vi "Begin.vi"(11 "Image Size":T1=enum."160x120") -> (0 "error out":errorcluster)   [LabVIEW 2011]
doc: "Called before other user functions, this VI is expected to open initial I/O refnums, load in file data, and do all program initialization. Notice that the <B>error out</B> terminal is simply used for data flow. Wiring it to other structures or subVIs ensures that this VI runs first."
uses:
  <vilib>/Rock Robotics/WPI/Camera/WPI_CameraImageSize.ctl
  <vilib>/Rock Robotics/WPI/Camera/WPI_CameraWhite Balance Values.ctl
  <vilib>/Rock Robotics/WPI/Camera/WPI_CameraExposure Values.ctl
  <vilib>/Rock Robotics/WPI/Camera/WPI_CameraFrameRate.ctl
  <vilib>/Rock Robotics/SystemInterfaces/DIO/FPGA_DIOPWMChannel.ctl
  <vilib>/Rock Robotics/SystemInterfaces/Typedef/FPGA_TypedefDigitalModule.ctl
  <vilib>/Rock Robotics/SystemInterfaces/Typedef/FPGA_TypedefAnalogModule.ctl
  <vilib>/Rock Robotics/SystemInterfaces/AI/FPGA_AIChannel.ctl
  <vilib>/Rock Robotics/SystemInterfaces/DIO/FPGA_DIOChannel.ctl
  <vilib>/Rock Robotics/SystemInterfaces/DIO/FPGA_DIORelayChannel.ctl
  <vilib>/Rock Robotics/WPI/Joystick/WPI_JoystickDeviceEnum.ctl
  <vilib>/Rock Robotics/WPI/Relay/WPI_RelayDirection.ctl
  <vilib>/Rock Robotics/SystemInterfaces/Typedef/FPGA_TypedefSolenoidModule.ctl
  <vilib>/Rock Robotics/WPI/Solenoid/WPI_SolenoidChannel.ctl
  <vilib>/Rock Robotics/WPI/RobotDrive/WPI_RobotDriveOpen4MotorWithVictor.vi
  <vilib>/Rock Robotics/WPI/MotorControl/WPI_MotorControlOpen Victor.vi
  <vilib>/Rock Robotics/WPI/Counter/WPI_CounterDigitalInputToDigitalSource.vi
  <vilib>/Rock Robotics/WPI/Counter/WPI_CounterOpen Gear Tooth Sensor Mode.vi
  <vilib>/Rock Robotics/WPI/Solenoid/WPI_SolenoidOpenDouble.vi
  <vilib>/Rock Robotics/WPI/Compressor/WPI_CompressorGetSetRefNum.vi
  <vilib>/Rock Robotics/WPI/Encoder/WPI_EncoderType.ctl
panel:
  in  "Image Size 2":T1=enum."160x120"
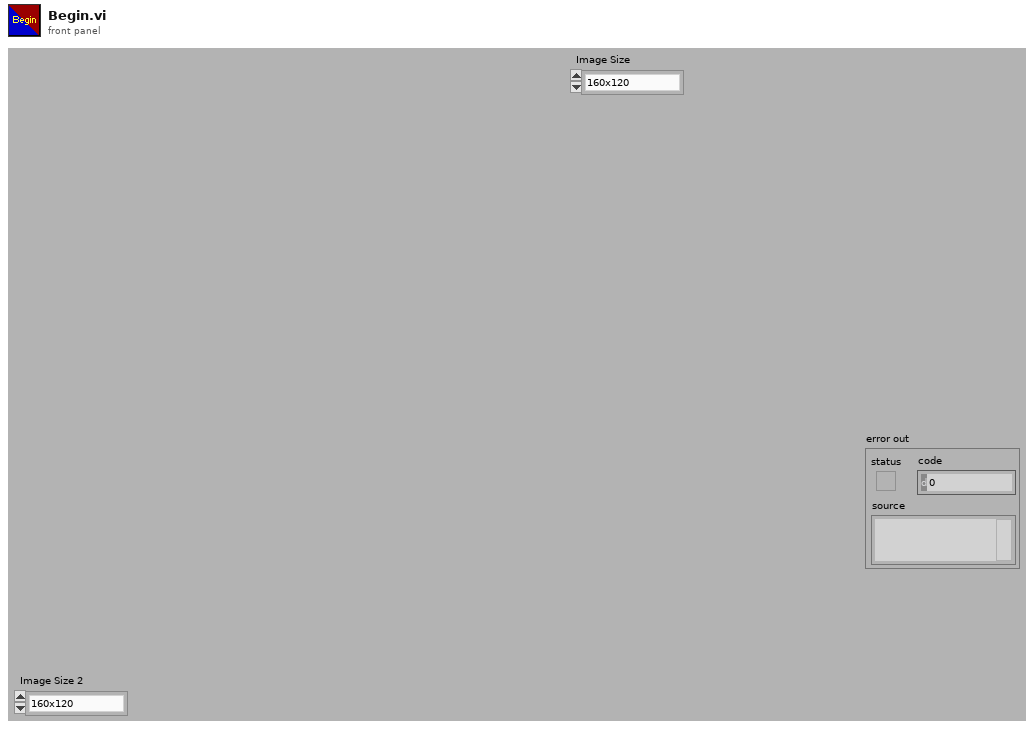
[diagram p1: front panel]
types:
  T1 = typedef "WPI_CameraImageSize.ctl" = enum16{"640x480", "320x240", "160x120"}
  T2 = typedef "FPGA_DIOChannel.ctl" = enum8{"DIO 1", "DIO 2", "DIO 3", "DIO 4", "DIO 5", "DIO 6", "DIO 7", "DIO 8", "DIO 9", "DIO 10", "DIO 11", "DIO 12", "DIO 13", "DIO 14", "Invalid"}
  T3 = typedef "FPGA_TypedefDigitalModule.ctl" = enum16{"Digital Module 1", "Digital Module 2"}
  T4 = typedef "WPI_RelayDirection.ctl" = enum16{"Both directions", "Forward only", "Reverse only"}
  T5 = typedef "FPGA_DIORelayChannel.ctl" = enum8{"Relay 1", "Relay 2", "Relay 3", "Relay 4", "Relay 5", "Relay 6", "Relay 7", "Relay 8", "Invalid"}
  T6 = typedef "WPI_SolenoidChannel.ctl" = enum8{"Solenoid 1", "Solenoid 2", "Solenoid 3", "Solenoid 4", "Solenoid 5", "Solenoid 6", "Solenoid 7", "Solenoid 8", "Invalid"}
  T7 = typedef "FPGA_TypedefSolenoidModule.ctl" = enum16{"Solenoid Module 1", "Solenoid Module 2"}
  T8 = typedef "WPI_JoystickDeviceEnum.ctl" = enum16{"USB 1", "USB 2", "USB 3", "USB 4", "Kinect 1", "Kinect 2"}
  T9 = typedef "FPGA_DIOPWMChannel.ctl" = enum8{"PWM 1", "PWM 2", "PWM 3", "PWM 4", "PWM 5", "PWM 6", "PWM 7", "PWM 8", "PWM 9", "PWM 10", "Invalid"}
  T10 = typedef "FPGA_AIChannel.ctl" = enum8{"AI 1", "AI 2", "AI 3", "AI 4", "AI 5", "AI 6", "AI 7", "AI 8", "Invalid"}
  T11 = typedef "FPGA_TypedefAnalogModule.ctl" = enum16{"Analog Module 1", "Analog Module 2"}
  T12 = typedef "WPI_CameraFrameRate.ctl" = u32
  T13 = typedef "WPI_CameraExposure Values.ctl" = enum16{"Auto", "Flicker-free 50 Hz", "Flicker-free 60 Hz", "Hold current"}
  T14 = typedef "WPI_CameraWhite Balance Values.ctl" = enum16{"Auto", "Fixed indoor", "Fixed outdoor 1", "Fixed outdoor 2", "Fixed fluorescent 1", "Fixed fluorescent 2", "Hold current"}
  T15 = typedef "WPI_MotorControlDeviceRef.ctl" = cluster{"DeviceStatus":errorcluster, "Type":enum16{"PWM", "CAN"}, "PWM":cluster{"Digital Module":T3, "PWM Channel":T9, "DeadBand":T16}, "CAN":cluster{"Device Number":u8, "Control Mode":T17, "Semaphore":T18, "Max Vout":dbl}, "Invert":bool, "TransformRef":T19, "InvTransformRef":T19}
  T16 = typedef "WPI_PWMDeadband.ctl" = cluster{"Name":string, "maxPositivePwm":i32, "minPositivePwm":i32, "centerPwm":i32, "maxNegativePwm":i32, "minNegativePwm":i32, "angularRange":u16}
  T17 = typedef "WPI_CANJaguar_ControlMode.ctl" = enum8{"Percent VBus", "Current", "Speed", "Position", "Voltage"}
  T18 = typedef "Semaphore RefNum" = refnum<k1>
  T19 = typedef "WPI_PWMTransform_ConPane.ctl" = refnum<vi>
  T20 = typedef "WPI_RobotDriveDevRef.ctl" = cluster{"DevStatus":errorcluster, "Motors[]":T15[], "Square Inputs":bool, "Max Output":dbl, "Isochronous":bool}
  T21 = typedef "WPI_CameraDevRef.ctl" = cluster{"Camera Address":string, "CameraStatus":errorcluster, "Acquire Image Notifier":refnum<notifier>}
  T22 = typedef "WPI_EncoderType.ctl" = enum16{"1x", "2x", "4x"}
  T23 = typedef "WPI_DigitalInputDevRef.ctl" = cluster{"DevStatus":errorcluster, "DIO Channel":T2, "Digital Module":T3}
  T24 = typedef "FPGA_CounterEncoderSourceConvertionLVSourceType.ctl" = cluster{"DevStatus":errorcluster, "AnalogTriggerMode?":bool, "DigitalMode":cluster{"Digital Module":T3, "DIO Channel":T25}, "AnalogTriggerMode":cluster{"AnalogTriggerIndex":T26, "OutputType":T27}}
  T25 = typedef "FPGA_DIODigitalSourceChannel.ctl" = enum8{"DIO 1", "DIO 2", "DIO 3", "DIO 4", "DIO 5", "DIO 6", "DIO 7", "DIO 8", "DIO 9", "DIO 10", "DIO 11", "DIO 12", "DIO 13", "DIO 14", "Disabled"}
  T26 = typedef "FPGA_AnalogTriggerIndex.ctl" = enum8{"Trig 0", "Trig 1", "Trig 2", "Trig 3", "Trig 4", "Trig 5", "Trig 6", "Trig 7", "Invalid"}
  T27 = typedef "FPGA_AnalogTriggerOutType.ctl" = enum16{"InWindow", "TriggerState", "Rising", "Falling"}
  T28 = typedef "WPI_EncoderDevRef.ctl" = cluster{"DevStatus":errorcluster, "EncoderIndex":T29, "CounterIndex":T30, "DistancePerCount":dbl, "Decoding Type":T22}
  T29 = typedef "FPGA_EncoderIdx.ctl" = enum8{"Enc 0", "Enc 1", "Enc 2", "Enc 3", "Invalid"}
  T30 = typedef "FPGA_CounterCtrSystemIndex.ctl" = enum8{"Ctr 0", "Ctr 1", "Ctr 2", "Ctr 3", "Ctr 4", "Ctr 5", "Ctr 6", "Ctr 7", "Invalid"}
  T31 = typedef "WPI_JoystickDevRef.ctl" = cluster{"Device":T8}
  T32 = typedef "WPI_AnalogChannelDevRef.ctl" = cluster{"DevStatus":errorcluster, "Analog Module":T11, "Analog Channel":T10}
  T33 = typedef "WPI_RelayDevRef.ctl" = cluster{"DevStatus":errorcluster, "Relay Channel":T5, "Digital Module":T3, "Relay Direction":T4}
  T34 = typedef "WPI_SolenoidDevRef.ctl" = cluster{"DevStatus":errorcluster, "Solenoid Module":T7, "Forward Solenoid Channel":T6, "Reverse Solenoid Channel":T6}
  T35 = typedef "WPI_CompressorDevRef.ctl" = cluster{"DevStatus":errorcluster, "DigitalInputDevRef":T23, "RelayDevRef":T33}
  T36 = typedef "WPI_CounterDevRef.ctl" = cluster{"DevStatus":errorcluster, "CntIndex":T30}
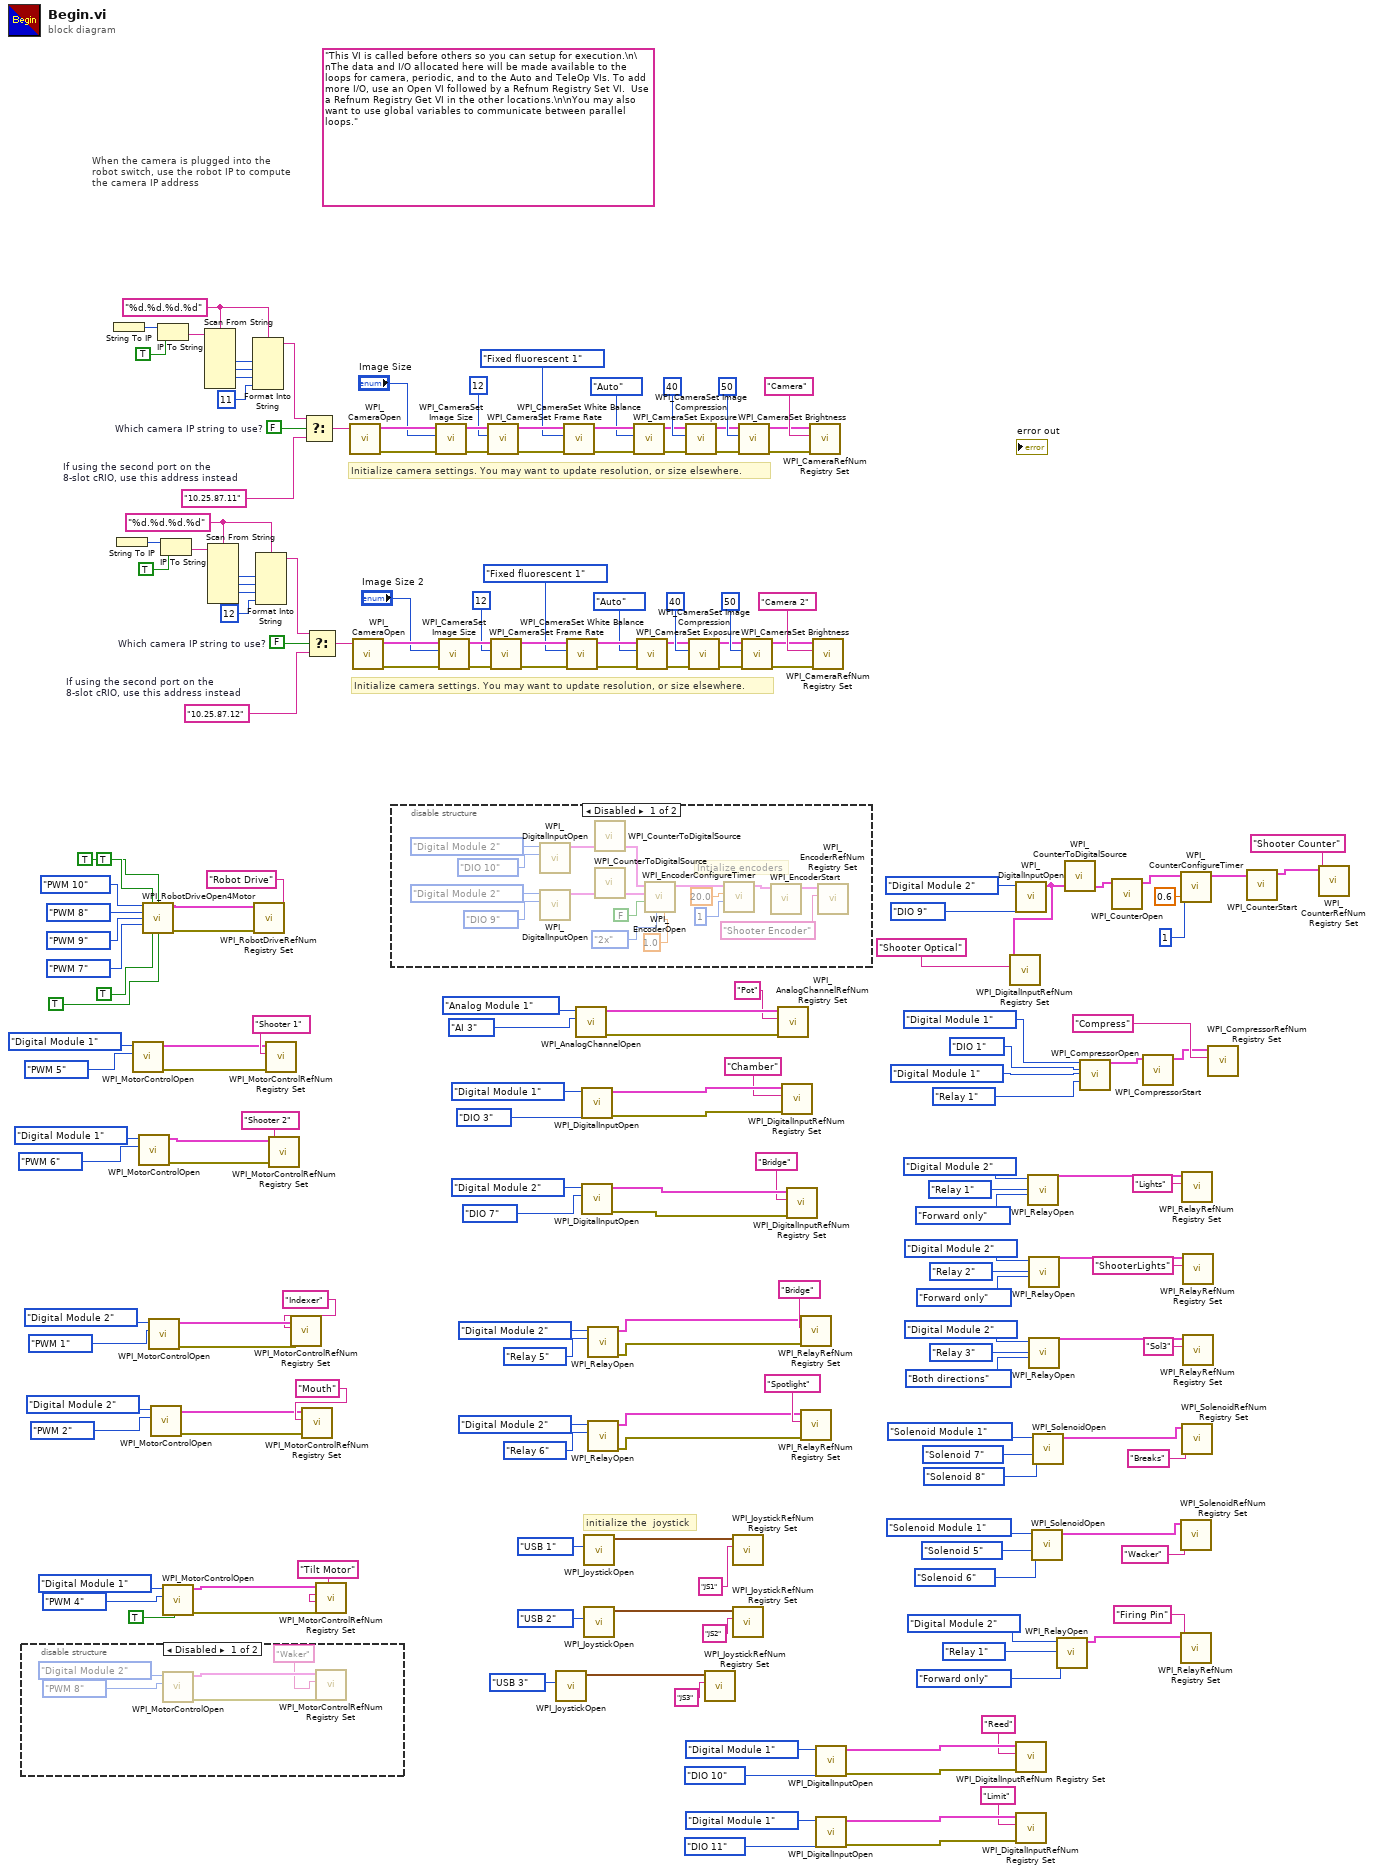
[diagram p0: block diagram]
diagram:
  w130 = FALSE  # Which camera IP string to use?
  w134 = "%d.%d.%d.%d" ("format string")
  w131 = "10.25.87.12"  # If using the second port on the 8-slot cRIO, use this address instead
  w163 = FALSE  # Which camera IP string to use?
  w167 = "%d.%d.%d.%d" ("format string")
  (unwired) "This VI is called before others so you can setup for execution.\n\nThe data and I/O allocated here will be made available to the loops for camera, periodic, and to the Auto and TeleOp VIs. To add more I/O, use an Open VI followed by a Refnum Registry Set VI.  Use a Refnum Registry Get VI in the other locations.\n\nYou may also want to use global variables to communicate between parallel loops."
  w164 = "10.25.87.11"  # If using the second port on the 8-slot cRIO, use this address instead
  # "initialize the  joystick"
  # "Initialize camera settings. You may want to update resolution, or size elsewhere."
  # "When the camera is plugged into the\nrobot switch, use the robot IP to compute\nthe camera IP address"
  # "Initialize camera settings. You may want to update resolution, or size elsewhere."
  n1 = disable-structure shown="Disabled" {
    frame Disabled {
      n2 = call-poly <vilib>:"WPI_MotorControlOpen.vi"("PWM Channel"=FPGA_DIOPWMChannel."PWM 8", "Digital Module (Module 1)"=FPGA_TypedefDigitalModule."Digital Module 2") -> ("error out"=w200:errorcluster, "MotorControlDeviceRef"=w199:T15)  [unwired: 8 in]
      n3 = call <vilib>:"WPI_MotorControlRefNum Registry Set.vi"("error in (no error)"=w200, "refnum name"="Waker", "MotorControlDevRef"=w199) -> ()  [unwired: 7 in, 2 out]
    }
    frame Enabled {
    }
  }
  n4 = String To IP() -> (0:w174:u32)  [unwired: 1 in]
  n5 = String To IP() -> (0:w141:u32)  [unwired: 1 in]
  n6 = call-poly <vilib>:"WPI_MotorControlOpen.vi"("PWM Channel"=FPGA_DIOPWMChannel."PWM 5", "Digital Module (Module 1)"=FPGA_TypedefDigitalModule."Digital Module 1") -> ("error out"=w113:errorcluster, "MotorControlDeviceRef"=w114:T15)  [unwired: 8 in]
  n7 = call-poly <vilib>:"WPI_MotorControlOpen.vi"("PWM Channel"=FPGA_DIOPWMChannel."PWM 6", "Digital Module (Module 1)"=FPGA_TypedefDigitalModule."Digital Module 1") -> ("error out"=w111:errorcluster, "MotorControlDeviceRef"=w112:T15)  [unwired: 8 in]
  n8 = call-poly <vilib>:"WPI_RobotDriveOpen4Motor.vi"("Rear Left Motor"=FPGA_DIOPWMChannel."PWM 10", "Rear Left Motor Inverted"=TRUE, "Rear Right Motor Inverted"=TRUE, "Rear Right Motor"=FPGA_DIOPWMChannel."PWM 8", "Front Left Motor"=FPGA_DIOPWMChannel."PWM 9", "Front Right Motor"=FPGA_DIOPWMChannel."PWM 7", "Front Left Motor Inverted"=TRUE, "Front Right Motor Inverted"=TRUE) -> ("RobotDriveDevRef"=w73:T20, "error out"=w72:errorcluster)  [unwired: 6 in]
  n9 = call-poly <vilib>:"WPI_MotorControlOpen.vi"("PWM Channel"=FPGA_DIOPWMChannel."PWM 1", "Digital Module (Module 1)"=FPGA_TypedefDigitalModule."Digital Module 2") -> ("error out"=w81:errorcluster, "MotorControlDeviceRef"=w82:T15)  [unwired: 8 in]
  n10 = call-poly <vilib>:"WPI_MotorControlOpen.vi"("PWM Channel"=FPGA_DIOPWMChannel."PWM 2", "Digital Module (Module 1)"=FPGA_TypedefDigitalModule."Digital Module 2") -> ("error out"=w106:errorcluster, "MotorControlDeviceRef"=w107:T15)  [unwired: 8 in]
  n11 = IP To String(1:TRUE ("dot notation? (F)"), 2:w174) -> (0:w172:string)
  n12 = IP To String(1:TRUE ("dot notation? (F)"), 2:w141) -> (0:w139:string)
  n13 = call-poly <vilib>:"WPI_MotorControlOpen.vi"("Invert"=TRUE, "PWM Channel"=FPGA_DIOPWMChannel."PWM 4", "Digital Module (Module 1)"=FPGA_TypedefDigitalModule."Digital Module 1") -> ("error out"=w100:errorcluster, "MotorControlDeviceRef"=w101:T15)  [unwired: 7 in]
  n14 = Scan From String(format string=w167, input string=w172) -> (output 1=w171:i32, output 2=w170:i32, output 3=w169:i32)  [unwired: 7 in, 3 out]
  n15 = Scan From String(format string=w134, input string=w139) -> (output 1=w138:i32, output 2=w137:i32, output 3=w136:i32)  [unwired: 7 in, 3 out]
  n16 = Format Into String(format string=w167, w171, w170, w169, 11 ("Compression")) -> (resulting string=w165:string)  [unwired: 2 in, 1 out]
  n17 = call <vilib>:"WPI_RobotDriveRefNum Registry Set.vi"("error in (no error)"=w72, "refnum name"="Robot Drive", "RobotDriveDevRef"=w73) -> ()  [unwired: 7 in, 2 out]
  n18 = Format Into String(format string=w134, w138, w137, w136, 12 ("Compression")) -> (resulting string=w132:string)  [unwired: 2 in, 1 out]
  n19 = call <vilib>:"WPI_MotorControlRefNum Registry Set.vi"("error in (no error)"=w113, "refnum name"="Shooter 1", "MotorControlDevRef"=w114) -> ()  [unwired: 7 in, 2 out]
  n20 = call <vilib>:"WPI_MotorControlRefNum Registry Set.vi"("error in (no error)"=w111, "refnum name"="Shooter 2", "MotorControlDevRef"=w112) -> ()  [unwired: 7 in, 2 out]
  n21 = call <vilib>:"WPI_MotorControlRefNum Registry Set.vi"("error in (no error)"=w81, "refnum name"="Indexer", "MotorControlDevRef"=w82) -> ()  [unwired: 7 in, 2 out]
  n22 = call <vilib>:"WPI_MotorControlRefNum Registry Set.vi"("error in (no error)"=w106, "refnum name"="Mouth", "MotorControlDevRef"=w107) -> ()  [unwired: 7 in, 2 out]
  n23 = Select(t=w165, s=w163, f=w164) -> (s? t:f=w166:string)
  n24 = Select(t=w132, s=w130, f=w131) -> (s? t:f=w133:string)
  n25 = call <vilib>:"WPI_MotorControlRefNum Registry Set.vi"("error in (no error)"=w100, "refnum name"="Tilt Motor", "MotorControlDevRef"=w101) -> ()  [unwired: 7 in, 2 out]
  n26 = call <vilib>:"WPI_CameraOpen.vi"("Camera Address"=w166) -> ("error out"=w186:errorcluster, "CameraDevRef"=w187:T21)  [unwired: 1 in, 8 out]
  n27 = call <vilib>:"WPI_CameraOpen.vi"("Camera Address"=w133) -> ("error out"=w153:errorcluster, "CameraDevRef"=w154:T21)  [unwired: 1 in, 8 out]
  n28 = disable-structure shown="Disabled" {
    frame Disabled {
      # "Intialize encoders"
      n29 = call <vilib>:"WPI_DigitalInputOpen.vi"("DIO Channel"=FPGA_DIOChannel."DIO 10", "Digital Module (Module 1)"=FPGA_TypedefDigitalModule."Digital Module 2") -> ("DigitalInputDevRef"=w215:T23)  [unwired: 8 in, 1 out]
      n30 = call <vilib>:"WPI_DigitalInputOpen.vi"("DIO Channel"=FPGA_DIOChannel."DIO 9", "Digital Module (Module 1)"=FPGA_TypedefDigitalModule."Digital Module 2") -> ("DigitalInputDevRef"=w211:T23)  [unwired: 8 in, 1 out]
      n31 = call-poly <vilib>:"WPI_CounterToDigitalSource.vi"("DigitalInputDevRef"=w215) -> ("Digital Source"=w214:T24)  [unwired: 6 in]
      n32 = call-poly <vilib>:"WPI_CounterToDigitalSource.vi"("DigitalInputDevRef"=w211) -> ("Digital Source"=w210:T24)  [unwired: 6 in]
      n33 = call <vilib>:"WPI_EncoderOpen.vi"("DistancePerCount"=1.0, "Decoding Type"=WPI_EncoderType."2x", "Invert Direction (False)"=FALSE, "BSource"=w210, "ASource"=w214) -> ("EncoderDevRef"=w208:T28)  [unwired: 5 in, 1 out]
      n34 = call <vilib>:"WPI_EncoderConfigureTimer.vi"("Number Samples to Average"=u8 1, "Minimum Rate"=20.0, "EncoderDevRef"=w208) -> ("EncoderDevRef"=w202:T28)  [unwired: 7 in, 1 out]
      n35 = call <vilib>:"WPI_EncoderStart.vi"("EncoderDevRef"=w202) -> ("EncoderDevRef"=w201:T28)  [unwired: 9 in, 1 out]
      n36 = call <vilib>:"WPI_EncoderRefNum Registry Set.vi"("refnum name"="Shooter Encoder", "EncoderDevRef"=w201) -> ()  [unwired: 8 in, 2 out]
    }
    frame Enabled {
    }
  }
  n37 = call <vilib>:"WPI_CameraSet Image Size.vi"("error in (no error)"=w186, "Image Size"="Image Size", "CameraDevRef"=w187) -> ("error out"=w185:errorcluster, "CameraDevRef Out"=w188:T21)  [unwired: 7 out]
  n38 = call <vilib>:"WPI_CameraSet Image Size.vi"("error in (no error)"=w153, "Image Size"="Image Size 2", "CameraDevRef"=w154) -> ("error out"=w152:errorcluster, "CameraDevRef Out"=w155:T21)  [unwired: 7 out]
  n39 = call <vilib>:"WPI_CameraSet Frame Rate.vi"("error in (no error)"=w185, "Frame Rate (fps)"=T12 12, "CameraDevRef"=w188) -> ("error out"=w184:errorcluster, "CameraDevRef Out"=w190:T21)  [unwired: 7 out]
  n40 = call <vilib>:"WPI_CameraSet Frame Rate.vi"("error in (no error)"=w152, "Frame Rate (fps)"=T12 12, "CameraDevRef"=w155) -> ("error out"=w151:errorcluster, "CameraDevRef Out"=w157:T21)  [unwired: 7 out]
  n41 = call <vilib>:"WPI_JoystickOpen.vi"("JoystickDevice"=WPI_JoystickDeviceEnum."USB 3") -> ("JoystickDevRef"=w50:T31)  [unwired: 10 out]
  n42 = call <vilib>:"WPI_CameraSet White Balance.vi"("error in (no error)"=w184, "White Balance"=WPI_CameraWhite_Balance_Values."Fixed fluorescent 1", "CameraDevRef"=w190) -> ("error out"=w183:errorcluster, "CameraDevRef Out"=w189:T21)  [unwired: 7 out]
  n43 = call <vilib>:"WPI_CameraSet White Balance.vi"("error in (no error)"=w151, "White Balance"=WPI_CameraWhite_Balance_Values."Fixed fluorescent 1", "CameraDevRef"=w157) -> ("error out"=w150:errorcluster, "CameraDevRef Out"=w156:T21)  [unwired: 7 out]
  n44 = call <vilib>:"WPI_AnalogChannelOpen.vi"("Analog Channel"=FPGA_AIChannel."AI 3", "Analog Module (Module 1)"=FPGA_TypedefAnalogModule."Analog Module 1") -> ("error out"=w95:errorcluster, "AIDeviceRef"=w97:T32)  [unwired: 8 in]
  n45 = call <vilib>:"WPI_DigitalInputOpen.vi"("DIO Channel"=FPGA_DIOChannel."DIO 3", "Digital Module (Module 1)"=FPGA_TypedefDigitalModule."Digital Module 1") -> ("error out"=w90:errorcluster, "DigitalInputDevRef"=w92:T23)  [unwired: 8 in]
  n46 = call <vilib>:"WPI_DigitalInputOpen.vi"("DIO Channel"=FPGA_DIOChannel."DIO 7", "Digital Module (Module 1)"=FPGA_TypedefDigitalModule."Digital Module 2") -> ("error out"=w62:errorcluster, "DigitalInputDevRef"=w64:T23)  [unwired: 8 in]
  n47 = call <vilib>:"WPI_JoystickOpen.vi"("JoystickDevice"=WPI_JoystickDeviceEnum."USB 1") -> ("JoystickDevRef"=w77:T31)  [unwired: 10 out]
  n48 = call <vilib>:"WPI_JoystickOpen.vi"("JoystickDevice"=WPI_JoystickDeviceEnum."USB 2") -> ("JoystickDevRef"=w76:T31)  [unwired: 10 out]
  n49 = call <vilib>:"WPI_RelayOpen.vi"("Relay Channel"=FPGA_DIORelayChannel."Relay 5", "Digital Module (Module 1)"=FPGA_TypedefDigitalModule."Digital Module 2") -> ("error out"=w67:errorcluster, "RelayDevRef"=w68:T33)  [unwired: 8 in]
  n50 = call <vilib>:"WPI_RelayOpen.vi"("Relay Channel"=FPGA_DIORelayChannel."Relay 6", "Digital Module (Module 1)"=FPGA_TypedefDigitalModule."Digital Module 2") -> ("error out"=w85:errorcluster, "RelayDevRef"=w86:T33)  [unwired: 8 in]
  n51 = call <vilib>:"WPI_CameraSet Exposure.vi"("error in (no error)"=w183, "Exposure"=WPI_CameraExposure_Values."Auto", "CameraDevRef"=w189) -> ("error out"=w182:errorcluster, "CameraDevRef Out"=w192:T21)  [unwired: 7 out]
  n52 = call <vilib>:"WPI_CameraSet Exposure.vi"("error in (no error)"=w150, "Exposure"=WPI_CameraExposure_Values."Auto", "CameraDevRef"=w156) -> ("error out"=w149:errorcluster, "CameraDevRef Out"=w159:T21)  [unwired: 7 out]
  n53 = call <vilib>:"WPI_CameraSet Image Compression.vi"("error in (no error)"=w182, "Compression"=40, "CameraDevRef"=w192) -> ("error out"=w181:errorcluster, "CameraDevRef Out"=w191:T21)  [unwired: 7 out]
  n54 = call <vilib>:"WPI_CameraSet Image Compression.vi"("error in (no error)"=w149, "Compression"=40, "CameraDevRef"=w159) -> ("error out"=w148:errorcluster, "CameraDevRef Out"=w158:T21)  [unwired: 7 out]
  n55 = call <vilib>:"WPI_JoystickRefNum Registry Set.vi"("refnum name"="JS3", "JoystickDevRef"=w50) -> ()  [unwired: 1 in, 9 out]
  n56 = call <vilib>:"WPI_JoystickRefNum Registry Set.vi"("refnum name"="JS1", "JoystickDevRef"=w77) -> ()  [unwired: 1 in, 9 out]
  n57 = call <vilib>:"WPI_JoystickRefNum Registry Set.vi"("refnum name"="JS2", "JoystickDevRef"=w76) -> ()  [unwired: 1 in, 9 out]
  n58 = call <vilib>:"WPI_CameraSet Brightness.vi"("error in (no error)"=w181, "Brightness"=50, "CameraDevRef"=w191) -> ("error out"=w179:errorcluster, "CameraDevRef Out"=w180:T21)  [unwired: 7 out]
  n59 = call <vilib>:"WPI_CameraSet Brightness.vi"("error in (no error)"=w148, "Brightness"=50, "CameraDevRef"=w158) -> ("error out"=w146:errorcluster, "CameraDevRef Out"=w147:T21)  [unwired: 7 out]
  n60 = call <vilib>:"WPI_AnalogChannelRefNum Registry Set.vi"("error in (no error)"=w95, "refnum name"="Pot", "AIDeviceRef"=w97) -> ()  [unwired: 7 in, 2 out]
  n61 = call <vilib>:"WPI_DigitalInputRefNum Registry Set.vi"("error in (no error)"=w90, "refnum name"="Chamber", "DigitalInputDevRef"=w92) -> ()  [unwired: 7 in, 2 out]
  n62 = call <vilib>:"WPI_DigitalInputRefNum Registry Set.vi"("error in (no error)"=w62, "refnum name"="Bridge", "DigitalInputDevRef"=w64) -> ()  [unwired: 7 in, 2 out]
  n63 = call <vilib>:"WPI_RelayRefNum Registry Set.vi"("error in (no error)"=w67, "refnum name"="Bridge", "RelayDevRef"=w68) -> ()  [unwired: 7 in, 2 out]
  n64 = call <vilib>:"WPI_RelayRefNum Registry Set.vi"("error in (no error)"=w85, "refnum name"="Spotlight", "RelayDevRef"=w86) -> ()  [unwired: 7 in, 2 out]
  n65 = call <vilib>:"WPI_CameraRefNum Registry Set.vi"("error in (no error)"=w179, "refnum name"="Camera", "CameraDevRef"=w180) -> ()  [unwired: 9 out]
  n66 = call <vilib>:"WPI_CameraRefNum Registry Set.vi"("error in (no error)"=w146, "refnum name"="Camera 2", "CameraDevRef"=w147) -> ()  [unwired: 9 out]
  n67 = call <vilib>:"WPI_DigitalInputOpen.vi"("DIO Channel"=FPGA_DIOChannel."DIO 10", "Digital Module (Module 1)"=FPGA_TypedefDigitalModule."Digital Module 1") -> ("error out"=w6:errorcluster, "DigitalInputDevRef"=w8:T23)  [unwired: 8 in]
  n68 = call <vilib>:"WPI_DigitalInputOpen.vi"("DIO Channel"=FPGA_DIOChannel."DIO 11", "Digital Module (Module 1)"=FPGA_TypedefDigitalModule."Digital Module 1") -> ("error out"=w1:errorcluster, "DigitalInputDevRef"=w3:T23)  [unwired: 8 in]
  n69 = call <vilib>:"WPI_DigitalInputOpen.vi"("DIO Channel"=FPGA_DIOChannel."DIO 9", "Digital Module (Module 1)"=FPGA_TypedefDigitalModule."Digital Module 2") -> ("DigitalInputDevRef"=w58:T23)  [unwired: 8 in, 1 out]
  n70 = call <vilib>:"WPI_DigitalInputRefNum Registry Set.vi"("refnum name"="Shooter Optical", "DigitalInputDevRef"=w58) -> ()  [unwired: 8 in, 2 out]
  n71 = call <vilib>:"WPI_DigitalInputRefNum Registry Set.vi"("error in (no error)"=w6, "refnum name"="Reed", "DigitalInputDevRef"=w8) -> ()  [unwired: 7 in, 2 out]
  n72 = call <vilib>:"WPI_DigitalInputRefNum Registry Set.vi"("error in (no error)"=w1, "refnum name"="Limit", "DigitalInputDevRef"=w3) -> ()  [unwired: 7 in, 2 out]
  n73 = call <vilib>:"WPI_RelayOpen.vi"("Relay Direction"=WPI_RelayDirection."Forward only", "Relay Channel"=FPGA_DIORelayChannel."Relay 1", "Digital Module (Module 1)"=FPGA_TypedefDigitalModule."Digital Module 2") -> ("RelayDevRef"=w42:T33)  [unwired: 7 in, 1 out]
  n74 = call <vilib>:"WPI_RelayOpen.vi"("Relay Direction"=WPI_RelayDirection."Forward only", "Relay Channel"=FPGA_DIORelayChannel."Relay 2", "Digital Module (Module 1)"=FPGA_TypedefDigitalModule."Digital Module 2") -> ("RelayDevRef"=w37:T33)  [unwired: 7 in, 1 out]
  n75 = call <vilib>:"WPI_RelayOpen.vi"("Relay Direction"=WPI_RelayDirection."Both directions", "Relay Channel"=FPGA_DIORelayChannel."Relay 3", "Digital Module (Module 1)"=FPGA_TypedefDigitalModule."Digital Module 2") -> ("RelayDevRef"=w32:T33)  [unwired: 7 in, 1 out]
  n76 = call-poly <vilib>:"WPI_SolenoidOpen.vi"("Reverse Solenoid Channel"=WPI_SolenoidChannel."Solenoid 6", "Forward Solenoid Channel"=WPI_SolenoidChannel."Solenoid 5", "Solenoid Module (Module 1)"=FPGA_TypedefSolenoidModule."Solenoid Module 1") -> ("SolenoidDevRef"=w20:T34)  [unwired: 7 in, 1 out]
  n77 = call-poly <vilib>:"WPI_SolenoidOpen.vi"("Reverse Solenoid Channel"=WPI_SolenoidChannel."Solenoid 8", "Forward Solenoid Channel"=WPI_SolenoidChannel."Solenoid 7", "Solenoid Module (Module 1)"=FPGA_TypedefSolenoidModule."Solenoid Module 1") -> ("SolenoidDevRef"=w25:T34)  [unwired: 7 in, 1 out]
  n78 = call <vilib>:"WPI_RelayOpen.vi"("Relay Direction"=WPI_RelayDirection."Forward only", "Relay Channel"=FPGA_DIORelayChannel."Relay 1", "Digital Module (Module 1)"=FPGA_TypedefDigitalModule."Digital Module 2") -> ("RelayDevRef"=w12:T33)  [unwired: 7 in, 1 out]
  n79 = call-poly <vilib>:"WPI_CounterToDigitalSource.vi"("DigitalInputDevRef"=w58) -> ("Digital Source"=w57:T24)  [unwired: 6 in]
  n80 = call <vilib>:"WPI_CompressorOpen.vi"("Pressure Switch Digital Module (Module 1)"=FPGA_TypedefDigitalModule."Digital Module 1", "Pressure Switch DIO Channel"=FPGA_DIOChannel."DIO 1", "Relay Digital Module (Module 1)"=FPGA_TypedefDigitalModule."Digital Module 1", "Relay Channel"=FPGA_DIORelayChannel."Relay 1") -> ("CompressorDevRef"=w16:T35)  [unwired: 10 in, 1 out]
  n81 = call-poly <vilib>:"WPI_CounterOpen.vi"("Source"=w57) -> ("CounterDevRef"=w53:T36)  [unwired: 9 in, 1 out]
  n82 = call <vilib>:"WPI_CompressorStart.vi"("CompressorDevRef"=w16) -> ("CompressorDevRef"=w17:T35)  [unwired: 9 in, 1 out]
  n83 = call <vilib>:"WPI_CounterConfigureTimer.vi"("Number Samples to Average"=u8 1, "MaxPeriod (sec)"=0.6, "CounterDevRef in"=w53) -> ("CounterDevRef out"=w55:T36)  [unwired: 7 in, 1 out]
  n84 = call <vilib>:"WPI_SolenoidRefNum Registry Set.vi"("refnum name"="Wacker", "SolenoidDevRef"=w20) -> ()  [unwired: 8 in, 2 out]
  n85 = call <vilib>:"WPI_RelayRefNum Registry Set.vi"("refnum name"="Firing Pin", "RelayDevRef"=w12) -> ()  [unwired: 8 in, 2 out]
  n86 = call <vilib>:"WPI_RelayRefNum Registry Set.vi"("refnum name"="Lights", "RelayDevRef"=w42) -> ()  [unwired: 8 in, 2 out]
  n87 = call <vilib>:"WPI_SolenoidRefNum Registry Set.vi"("refnum name"="Breaks", "SolenoidDevRef"=w25) -> ()  [unwired: 8 in, 2 out]
  n88 = call <vilib>:"WPI_RelayRefNum Registry Set.vi"("refnum name"="ShooterLights", "RelayDevRef"=w37) -> ()  [unwired: 8 in, 2 out]
  n89 = call <vilib>:"WPI_RelayRefNum Registry Set.vi"("refnum name"="Sol3", "RelayDevRef"=w32) -> ()  [unwired: 8 in, 2 out]
  n90 = call <vilib>:"WPI_CompressorRefNum Registry Set.vi"("refnum name"="Compress", "CompressorDevRef"=w17) -> ()  [unwired: 8 in, 2 out]
  n91 = call <vilib>:"WPI_CounterStart.vi"("CounterDevRef in"=w55) -> ("CounterDevRef out"=w54:T36)  [unwired: 9 in, 1 out]
  n92 = call <vilib>:"WPI_CounterRefNum Registry Set.vi"("refnum name"="Shooter Counter", "CounterDevRef"=w54) -> ()  [unwired: 8 in, 2 out]
